vi "Untitled 1.vi"() -> ()   [LabVIEW 2024]
uses:
  <vilib>/httpClient/ClientHandle.ctl
  <vilib>/httpClient/LabVIEWHTTPClient.lvlib
panel:
  in  "stop":bool
  in  "client handle out":T1
  in  "Cluster":T2={"name"="172.20.10.13", "error in (no error)"={"status"=FALSE, "code"=0, "source"=""}, "username"="iPhone di Luca", "Password"="iPhone di Luca"}
  out "error out":errorcluster
  in  "password":string="letizia16"
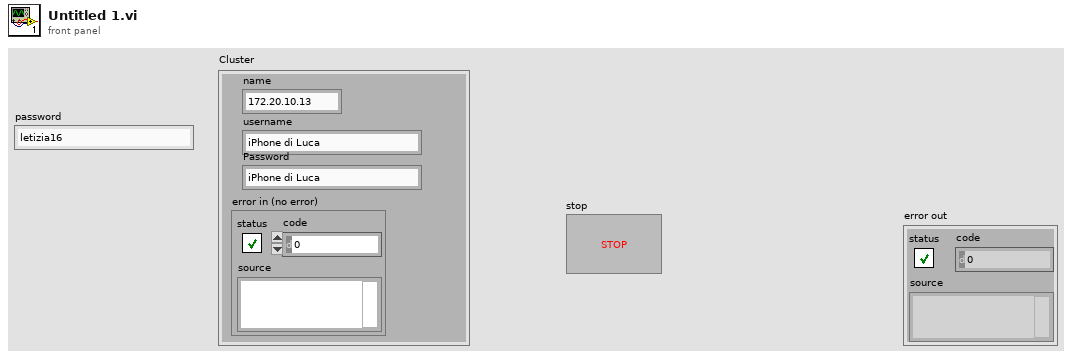
[diagram p1: front panel]
types:
  T1 = typedef "LabVIEWHTTPClient.lvlib/ClientHandle.ctl" = refnum<k1>
  T2 = cluster{"name":string, "error in (no error)":errorcluster, "username":string, "Password":string}
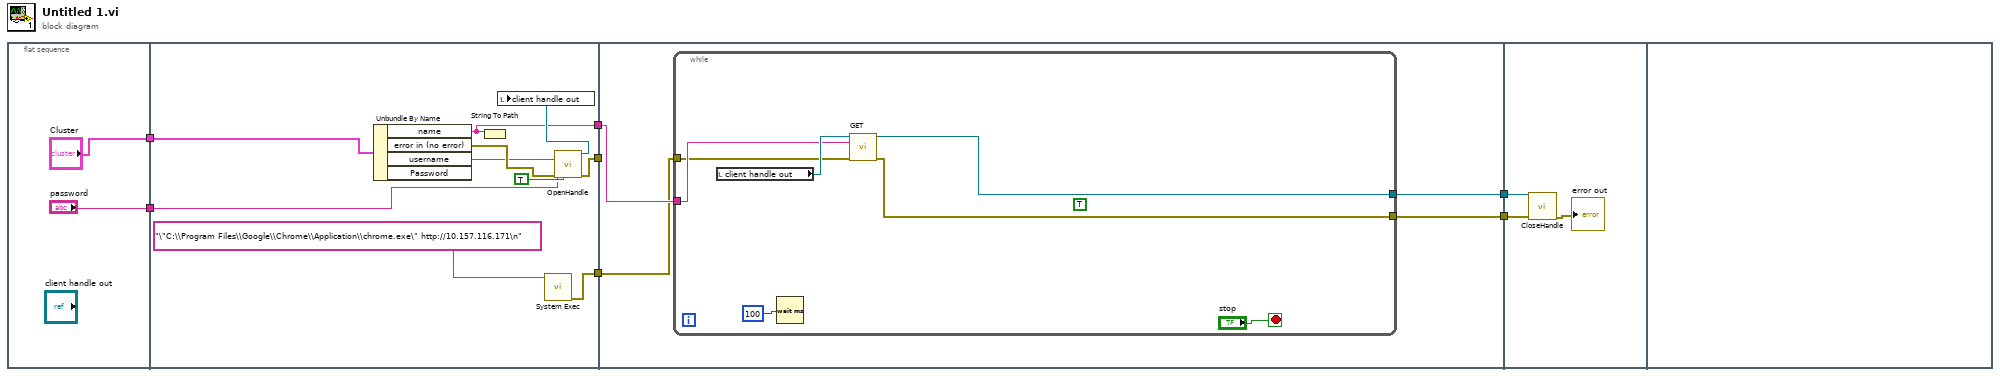
[diagram p0: block diagram]
diagram:
  n1 = flat-sequence {
    tunnel: ["Cluster"] -> w7
    tunnel: ["password"] -> w6
    tunnel: w7 -> [w18]
    tunnel: w6 -> [w14]
    tunnel: [w13] -> w5
    tunnel: [w12] -> w2
    tunnel: [w11] -> w1
    tunnel: w5 -> [w23]
    tunnel: [w22] -> w4
    tunnel: [w21] -> w3
    tunnel: w2 -> [_]
    tunnel: w1 -> [w20]
    tunnel: w4 -> [w32]
    tunnel: w3 -> [w31]
    frame #0 {
    }
    frame #1 {
      n2 = Unbundle By Name(w18) -> ("name"=w13:string, "error in (no error)"=w17:errorcluster, "username"=w16:string)  [unwired: 1 out]
      n3 = String To Path(string=w13) -> ()  [unwired: 1 out]
      n4 = call <vilib>:"System Exec.vi"("command line"="\"C:\\Program Files\\Google\\Chrome\\Application\\chrome.exe\" http://10.157.116.171\n") -> ("error out"=w11:errorcluster)  [unwired: 7 in, 3 out]
      n5 = call <vilib>:"OpenHandle.vi"("username"=w16, "password"=w14, "error in (no error)"=w17, "verify server(true)"=TRUE) -> ("client handle out"=w15:T1, "error out"=w12:errorcluster)  [unwired: 10 in]
      n6 = local write "client handle out"(w15) -> ()
    }
    frame #2 {
      n7 = while {
        tunnel: w23 -> [w29]
        tunnel: [w28] -> w21
        tunnel: [w24] -> w22
        tunnel: w20 -> [w25]
        stop <- "stop" stop-if-true
        (unwired) TRUE ("prepend array or string size? (T)")
        n8 = local read "client handle out"() -> (w30:T1)
        n9 = Wait (ms)(milliseconds to wait=u32 100) -> ()  [unwired: 1 out]
        n10 = call <vilib>:"GET.vi"("client handle"=w30, "url"=w29, "error in (no error)"=w25) -> ("client handle out"=w28:T1, "error out"=w24:errorcluster)  [unwired: 9 in, 2 out]
      }
    }
    frame #3 {
      n11 = call <vilib>:"CloseHandle.vi"("client handle"=w31, "error in (no error)"=w32) -> ("error out"=→"error out":errorcluster)  [unwired: 13 in]
    }
    frame #4 {
    }
  }
